vi "AUTON_Index.vi"(0 "Auton Array":dbl[][](array[numeric]), 5 "MeasuredHeading":dbl, 7 "LeftEncoder":dbl, 9 "RightEncoder":dbl) -> (4 "Right Drive":dbl, 6 "Left Drive":dbl, 8 "Shooter Elevation":dbl, 10 "Shooter Wheel F":dbl, 15 "Shooter Wheel B":dbl)   [LabVIEW 2012]
uses:
  Robot Global Data.vi
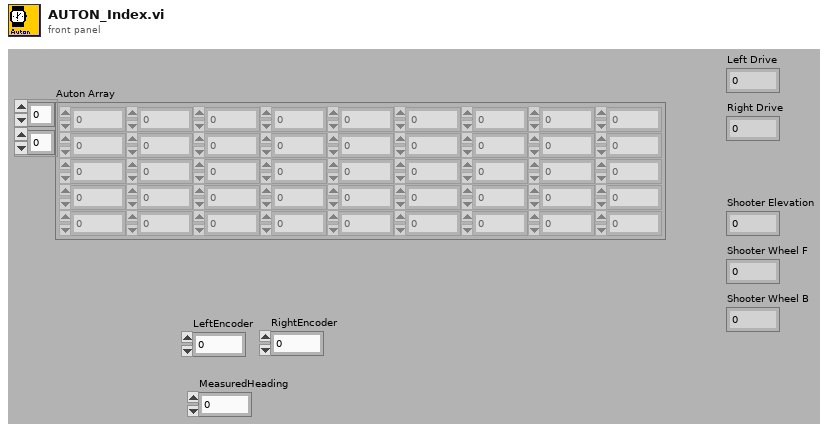
[diagram p1: front panel]
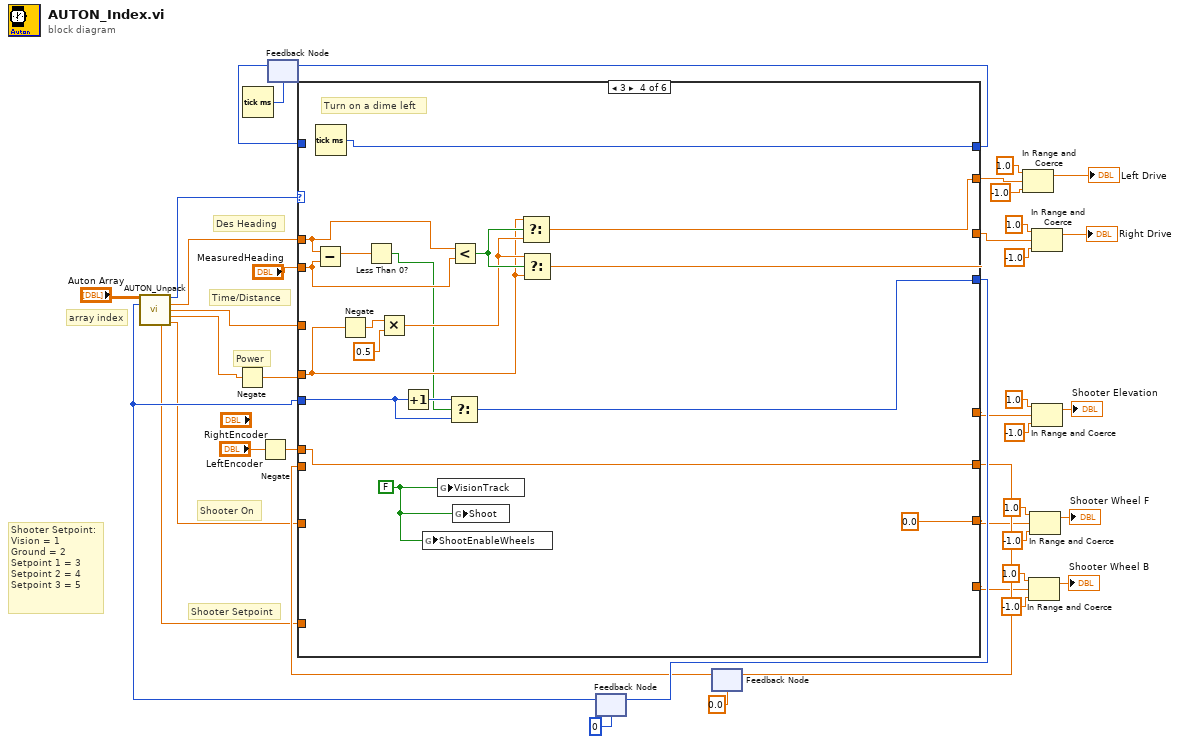
[diagram p0: block diagram]
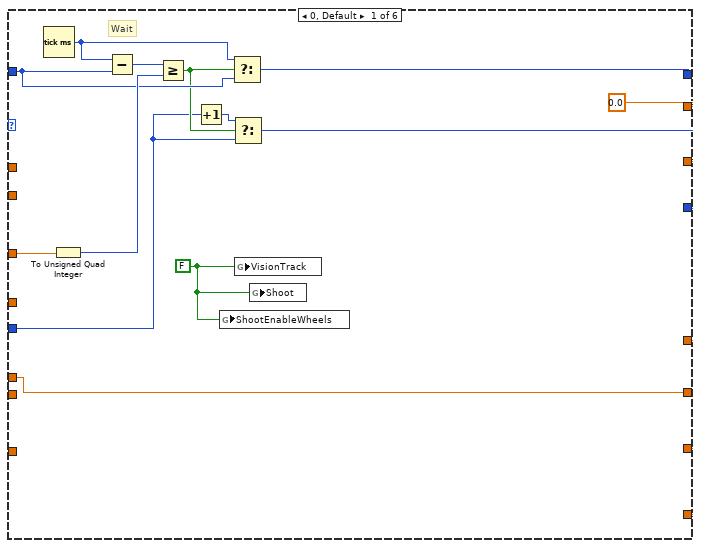
[diagram p2: hidden frame]
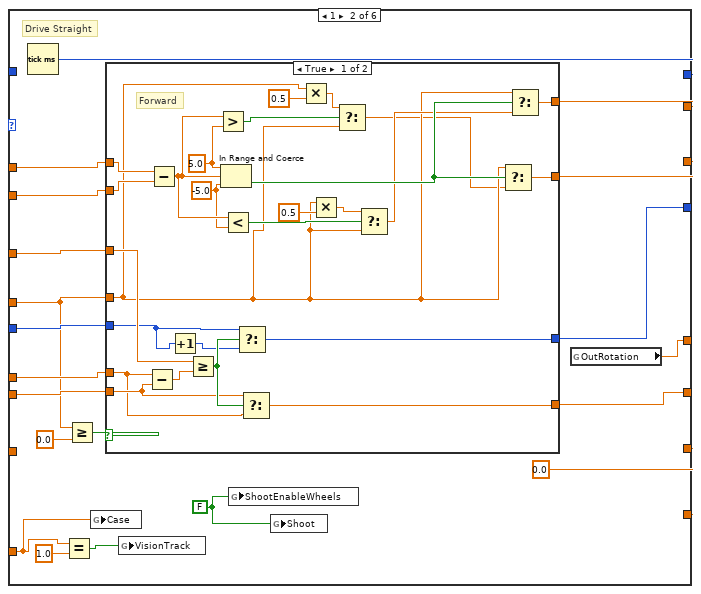
[diagram p3: hidden frame]
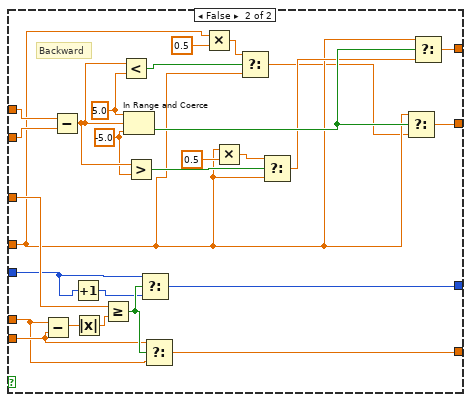
[diagram p4: hidden frame]
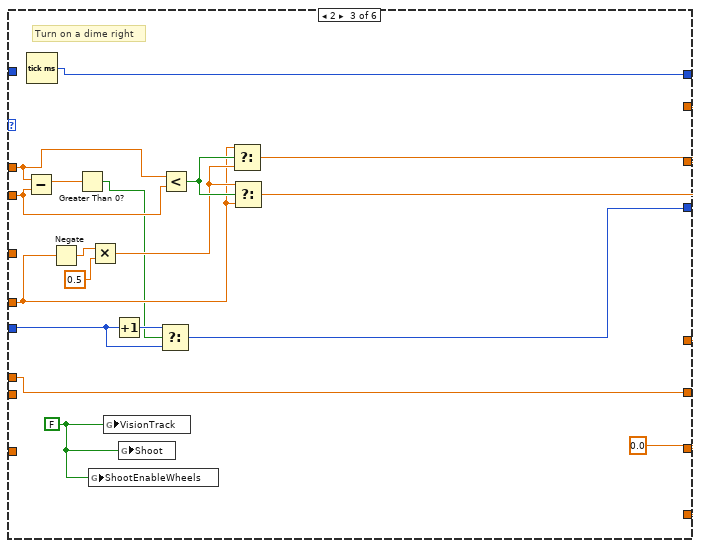
[diagram p5: hidden frame]
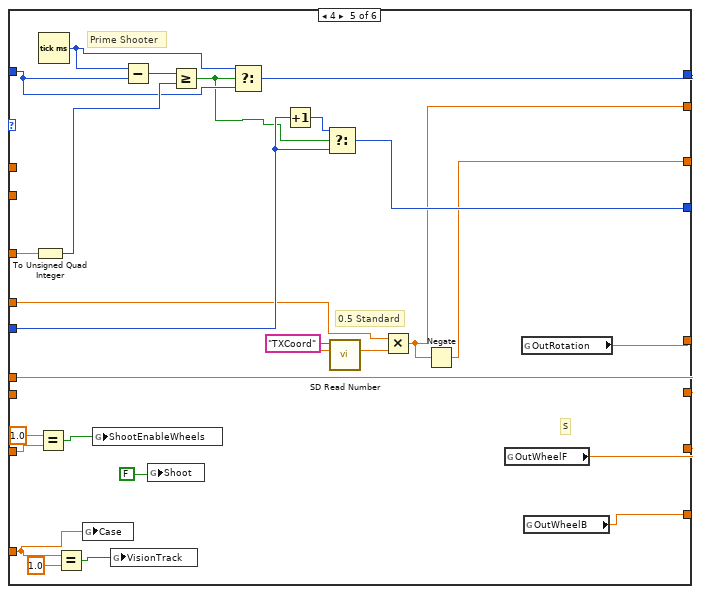
[diagram p6: hidden frame]
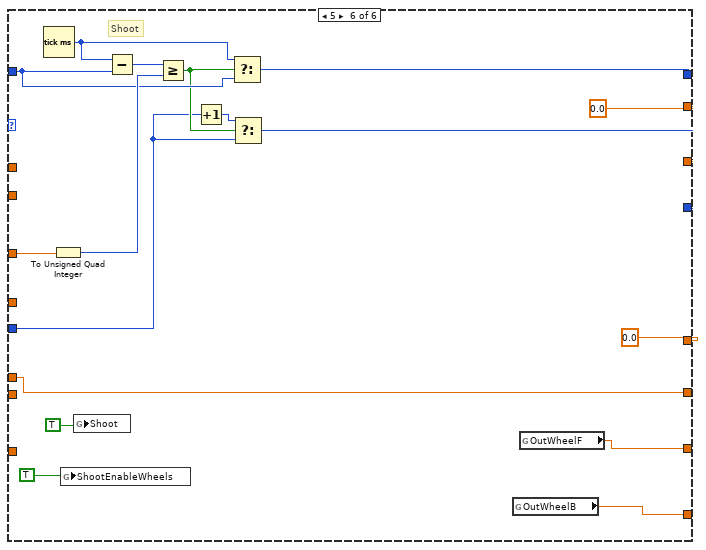
[diagram p7: hidden frame]
diagram:
  # "Shooter Setpoint:\nVision = 1\nGround = 2\nSetpoint 1 = 3\nSetpoint 2 = 4\nSetpoint 3 = 5"
  # "Shooter On"
  # "Shooter Setpoint"
  # "Des Heading"
  # "Time/Distance"
  # "Power"
  # "array index"
  n1 = Tick Count (ms)() -> (millisecond timer value=w38:u32)
  n2 = Negate(x="LeftEncoder") -> (-x=w1:dbl)
  n3 = feedback #1(w38) -> (w39:u32)
  n4 = feedback #2(0) -> (w19:i32)
  n5 = call "AUTON_Unpack.vi"("all rows"="Auton Array", "Index"=w19) -> ("Primitive ID"=w22:i16, "Desired Heading"=w21:dbl, "Time/Distance"=w20:dbl, "Power"=w4:dbl, "Shooter Case"=w5:dbl, "Shooter On"=w18:dbl)  [unwired: 6 in, 2 out]
  n6 = Negate(x=w4) -> (-x=w3:dbl)
  n7 = feedback #3(0.0) -> (w24:dbl)
  n8 = case shown="3" w22 {
    tunnel: [w45 w71 w139 w157 w187 w197] -> w26
    tunnel: w19 -> [w46 w66 w142 w160 w178 w198]
    tunnel: [w53 w63 w144 w162 w176 w205] -> w28
    tunnel: w39 -> [w50 _ _ _ w177 w202]
    tunnel: w20 -> [w44 w72 _ _ w179 w196]
    tunnel: w21 -> [_ w70 w137 w155 _ _]
    tunnel: [w41 w68 w140 w158 w172 w195] -> w36
    tunnel: [w41 w67 w141 w159 w171 w195] -> w29
    tunnel: w3 -> [_ w62 w131 w149 w173 _]
    tunnel: w1 -> [w42 w64 w138 w156 w188 w193]
    tunnel: "MeasuredHeading" -> [_ w69 w136 w154 _ _]
    tunnel: w24 -> [_ w65 _ _ _ _]
    tunnel: [w42 w73 w138 w156 w188 w193] -> w23
    tunnel: w18 -> [_ _ _ _ w169 _]
    tunnel: w5 -> [_ w56 _ _ w183 _]
    tunnel: [w41 w54 w128 w145 w165 w189] -> w8
    tunnel: [w41 w54 w128 w145 w166 w190] -> w7
    tunnel: [w41 w55 w128 w145 w175 0.0 ("ShootOutElev")] -> w6
    frame 0, Default {
      w43 = FALSE ("ShootTrackEnable")
      w41 = 0.0 ("Numeric")
      # "Wait"
      n9 = Tick Count (ms)() -> (millisecond timer value=w49:u32)
      n10 = To Unsigned Quad Integer(1:w44) -> (0:w51:u64)
      n11 = Subtract(x=w49, y=w50) -> (x-y=w52:u32)
      n12 = Greater Or Equal?(x=w52, y=w51) -> (x >= y?=w48:bool)
      n13 = Increment(x=w46) -> (x+1=w47:i32)
      n14 = global write "Robot Global Data.vi" "ShootEnableWheels"(w43) -> ()
      n15 = Select(t=w49, s=w48, f=w50) -> (s? t:f=w53:u32)
      n16 = Select(t=w47, s=w48, f=w46) -> (s? t:f=w45:i32)
      n17 = global write "Robot Global Data.vi" "VisionTrack"(w43) -> ()
      n18 = global write "Robot Global Data.vi" "Shoot"(w43) -> ()
    }
    frame 1 {
      w59 = FALSE ("ShootTrackEnable")
      w54 = 0.0 ("Numeric")
      # "Drive Straight"
      n19 = Tick Count (ms)() -> (millisecond timer value=w63:u32)
      n20 = Equal?(x=w56, y=1.0) -> (x = y?=w57:bool)
      n21 = Greater Or Equal?(x=w62, y=0.0) -> (x >= y?=w60:bool)
      n22 = global write "Robot Global Data.vi" "Case"(w56) -> ()
      n23 = case shown="True" w60 {
        tunnel: [w99 w126] -> w73
        tunnel: w72 -> [w97 w125]
        tunnel: [w95 w123] -> w71
        tunnel: w70 -> [w94 w122]
        tunnel: w69 -> [w93 w121]
        tunnel: [w91 w119] -> w68
        tunnel: [w90 w118] -> w67
        tunnel: w62 -> [w79 w107]
        tunnel: w66 -> [w76 w104]
        tunnel: w65 -> [w75 w103]
        tunnel: w64 -> [w74 w102]
        frame True {
          w87 = -5.0 ("lower limit")
          w89 = 5.0 ("upper limit")
          # "Forward"
          n24 = Subtract(x=w74, y=w75) -> (x-y=w98:dbl)
          n25 = Subtract(x=w94, y=w93) -> (x-y=w88:dbl)
          n26 = Increment(x=w76) -> (x+1=w77:i32)
          n27 = Greater Or Equal?(x=w97, y=w98) -> (x >= y?=w96:bool)
          n28 = Greater?(x=w88, y=w89) -> (0:w82:bool)
          n29 = In Range and Coerce(upper limit=w89, x=w88, lower limit=w87) -> (In Range?=w92:bool)  [unwired: 1 out]
          n30 = Less?(x=w88, y=w87) -> (x < y?=w86:bool)
          n31 = Select(t=w76, s=w96, f=w77) -> (s? t:f=w95:i32)
          n32 = Select(t=w75, s=w96, f=w74) -> (s? t:f=w99:dbl)
          n33 = Multiply(x=w79, y=0.5) -> (x*y=w81:dbl)
          n34 = Multiply(x=w79, y=0.5) -> (x*y=w84:dbl)
          n35 = Select(t=w81, s=w82, f=w79) -> (s? t:f=w78:dbl)
          n36 = Select(t=w84, s=w86, f=w79) -> (s? t:f=w83:dbl)
          n37 = Select(t=w79, s=w92, f=w78) -> (s? t:f=w90:dbl)
          n38 = Select(t=w79, s=w92, f=w83) -> (s? t:f=w91:dbl)
        }
        frame False {
          w115 = -5.0 ("lower limit")
          w117 = 5.0 ("upper limit")
          # "Backward"
          n39 = Subtract(x=w102, y=w103) -> (x-y=w100:dbl)
          n40 = Subtract(x=w122, y=w121) -> (x-y=w116:dbl)
          n41 = Increment(x=w104) -> (x+1=w105:i32)
          n42 = Absolute Value(x=w100) -> (abs(x)=w101:dbl)
          n43 = Greater Or Equal?(x=w125, y=w101) -> (x >= y?=w124:bool)
          n44 = Less?(x=w116, y=w117) -> (x < y?=w110:bool)
          n45 = In Range and Coerce(upper limit=w117, x=w116, lower limit=w115) -> (In Range?=w120:bool)  [unwired: 1 out]
          n46 = Greater?(x=w116, y=w115) -> (0:w114:bool)
          n47 = Select(t=w104, s=w124, f=w105) -> (s? t:f=w123:i32)
          n48 = Select(t=w103, s=w124, f=w102) -> (s? t:f=w126:dbl)
          n49 = Multiply(x=w107, y=0.5) -> (x*y=w109:dbl)
          n50 = Multiply(x=w107, y=0.5) -> (x*y=w112:dbl)
          n51 = Select(t=w109, s=w110, f=w107) -> (s? t:f=w106:dbl)
          n52 = Select(t=w112, s=w114, f=w107) -> (s? t:f=w111:dbl)
          n53 = Select(t=w107, s=w120, f=w106) -> (s? t:f=w118:dbl)
          n54 = Select(t=w107, s=w120, f=w111) -> (s? t:f=w119:dbl)
        }
      }
      n55 = global write "Robot Global Data.vi" "VisionTrack"(w57) -> ()
      n56 = global write "Robot Global Data.vi" "ShootEnableWheels"(w59) -> ()
      n57 = global write "Robot Global Data.vi" "Shoot"(w59) -> ()
      n58 = global read "Robot Global Data.vi" "OutRotation"() -> (w55:dbl)
    }
    frame 2 {
      w127 = FALSE ("ShootTrackEnable")
      w128 = 0.0 ("Numeric")
      # "Turn on a dime right"
      n59 = Subtract(x=w137, y=w136) -> (x-y=w130:dbl)
      n60 = Tick Count (ms)() -> (millisecond timer value=w144:u32)
      n61 = Negate(x=w131) -> (-x=w134:dbl)
      n62 = Greater Than 0?(x=w130) -> (x > 0?=w129:bool)
      n63 = global write "Robot Global Data.vi" "ShootEnableWheels"(w127) -> ()
      n64 = Multiply(x=w134, y=0.5) -> (x*y=w132:dbl)
      n65 = global write "Robot Global Data.vi" "VisionTrack"(w127) -> ()
      n66 = Increment(x=w142) -> (x+1=w143:i32)
      n67 = global write "Robot Global Data.vi" "Shoot"(w127) -> ()
      n68 = Select(t=w143, s=w129, f=w142) -> (s? t:f=w139:i32)
      n69 = Less?(x=w137, y=w136) -> (x < y?=w135:bool)
      n70 = Select(t=w131, s=w135, f=w132) -> (s? t:f=w140:dbl)
      n71 = Select(t=w132, s=w135, f=w131) -> (s? t:f=w141:dbl)
    }
    frame 3 {
      w146 = FALSE ("ShootTrackEnable")
      w145 = 0.0 ("Numeric")
      # "Turn on a dime left"
      n72 = Subtract(x=w155, y=w154) -> (x-y=w148:dbl)
      n73 = Tick Count (ms)() -> (millisecond timer value=w162:u32)
      n74 = Negate(x=w149) -> (-x=w152:dbl)
      n75 = Less Than 0?(x=w148) -> (x < 0?=w147:bool)
      n76 = Multiply(x=w152, y=0.5) -> (x*y=w150:dbl)
      n77 = Increment(x=w160) -> (x+1=w161:i32)
      n78 = global write "Robot Global Data.vi" "ShootEnableWheels"(w146) -> ()
      n79 = global write "Robot Global Data.vi" "VisionTrack"(w146) -> ()
      n80 = Select(t=w161, s=w147, f=w160) -> (s? t:f=w157:i32)
      n81 = Less?(x=w155, y=w154) -> (x < y?=w153:bool)
      n82 = global write "Robot Global Data.vi" "Shoot"(w146) -> ()
      n83 = Select(t=w149, s=w153, f=w150) -> (s? t:f=w158:dbl)
      n84 = Select(t=w150, s=w153, f=w149) -> (s? t:f=w159:dbl)
    }
    frame 4 {
      # "S"
      # "0.5 Standard"
      # "Prime Shooter"
      n85 = To Unsigned Quad Integer(1:w179) -> (0:w181:u64)
      n86 = Equal?(x=1.0, y=w169) -> (x = y?=w167:bool)
      n87 = Tick Count (ms)() -> (millisecond timer value=w180:u32)
      n88 = Equal?(x=w183, y=1.0) -> (x = y?=w184:bool)
      n89 = global write "Robot Global Data.vi" "Case"(w183) -> ()
      n90 = global write "Robot Global Data.vi" "ShootEnableWheels"(w167) -> ()
      n91 = global write "Robot Global Data.vi" "VisionTrack"(w184) -> ()
      n92 = Subtract(x=w180, y=w177) -> (x-y=w182:u32)
      n93 = global write "Robot Global Data.vi" "Shoot"(FALSE ("Shoot")) -> ()
      n94 = Greater Or Equal?(x=w182, y=w181) -> (x >= y?=w174:bool)
      n95 = Select(t=w180, s=w174, f=w177) -> (s? t:f=w176:u32)
      n96 = Increment(x=w178) -> (x+1=w186:i32)
      n97 = Select(t=w186, s=w174, f=w178) -> (s? t:f=w187:i32)
      n98 = call <vilib>:"SD Read Number.vi"("Name"="TXCoord") -> ("Numeric"=w163:dbl)  [unwired: 8 in, 2 out]
      n99 = Multiply(x=w173, y=w163) -> (x*y=w172:dbl)
      n100 = Negate(x=w172) -> (-x=w171:dbl)
      n101 = global read "Robot Global Data.vi" "OutWheelF"() -> (w166:dbl)
      n102 = global read "Robot Global Data.vi" "OutRotation"() -> (w175:dbl)
      n103 = global read "Robot Global Data.vi" "OutWheelB"() -> (w165:dbl)
    }
    frame 5 {
      w195 = 0.0 ("Numeric")
      # "Shoot"
      n104 = Tick Count (ms)() -> (millisecond timer value=w201:u32)
      n105 = To Unsigned Quad Integer(1:w196) -> (0:w203:u64)
      n106 = global write "Robot Global Data.vi" "ShootEnableWheels"(TRUE ("ShootEnableWheels")) -> ()
      n107 = global write "Robot Global Data.vi" "Shoot"(TRUE ("Shoot")) -> ()
      n108 = Subtract(x=w201, y=w202) -> (x-y=w204:u32)
      n109 = Greater Or Equal?(x=w204, y=w203) -> (x >= y?=w200:bool)
      n110 = Increment(x=w198) -> (x+1=w199:i32)
      n111 = Select(t=w201, s=w200, f=w202) -> (s? t:f=w205:u32)
      n112 = Select(t=w199, s=w200, f=w198) -> (s? t:f=w197:i32)
      n113 = global read "Robot Global Data.vi" "OutWheelB"() -> (w189:dbl)
      n114 = global read "Robot Global Data.vi" "OutWheelF"() -> (w190:dbl)
    }
  }
  n115 = feedback-in #1(w28) -> ()
  n116 = feedback-in #2(w26) -> ()
  n117 = feedback-in #3(w23) -> ()
  n118 = In Range and Coerce(upper limit=1.0, x=w36, lower limit=-1.0) -> (coerced(x)=→"Left Drive":dbl)  [unwired: 1 out]
  n119 = In Range and Coerce(upper limit=1.0, x=w8, lower limit=-1.0) -> (coerced(x)=→"Shooter Wheel B":dbl)  [unwired: 1 out]
  n120 = In Range and Coerce(upper limit=1.0, x=w7, lower limit=-1.0) -> (coerced(x)=→"Shooter Wheel F":dbl)  [unwired: 1 out]
  n121 = In Range and Coerce(upper limit=1.0, x=w29, lower limit=-1.0) -> (coerced(x)=→"Right Drive":dbl)  [unwired: 1 out]
  n122 = In Range and Coerce(upper limit=1.0, x=w6, lower limit=-1.0) -> (coerced(x)=→"Shooter Elevation":dbl)  [unwired: 1 out]
